vi "User jsObject.vi"(7 "DB Connection Ref":T1, 8 "error in (no error)":errorcluster, 9 "User Record (empty)":T2, 10 "User jsObject Name (\"USER\")":string="USER", 11 "Previous String (\"\")":string) -> (0 "error out":errorcluster, 2 "User Literal Object":string, 3 "User jsObject":string, 5 "User jsObject Definition":string)   [LabVIEW 2011]
uses:
  User Record.ctl
  SI.LIB/ODBC/SQL Controls/Connection Refnum.ctl
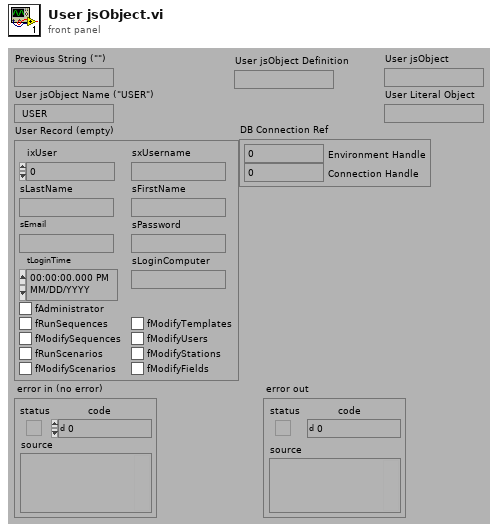
[diagram p1: front panel]
types:
  T1 = typedef "Connection Refnum.ctl" = cluster{"Environment Handle":i32, "Connection Handle":i32}
  T2 = typedef "User Record.ctl" = cluster{"ixUser":i32, "sxUsername":string, "sLastName":string, "sFirstName":string, "sEmail":string, "sPassword":string, "tLoginTime":timestamp, "sLoginComputer":string, "fAdministrator":bool, "fRunSequences":bool, "fModifySequences":bool, "fRunScenarios":bool, "fModifyScenarios":bool, "fModifyTemplates":bool, "fModifyUsers":bool, "fModifyStations":bool, "fModifyFields":bool}
  T3 = typedef "Station Record.ctl" = cluster{"ixStation":i32, "sxStationId":string, "sIP":string, "fVerified":bool}
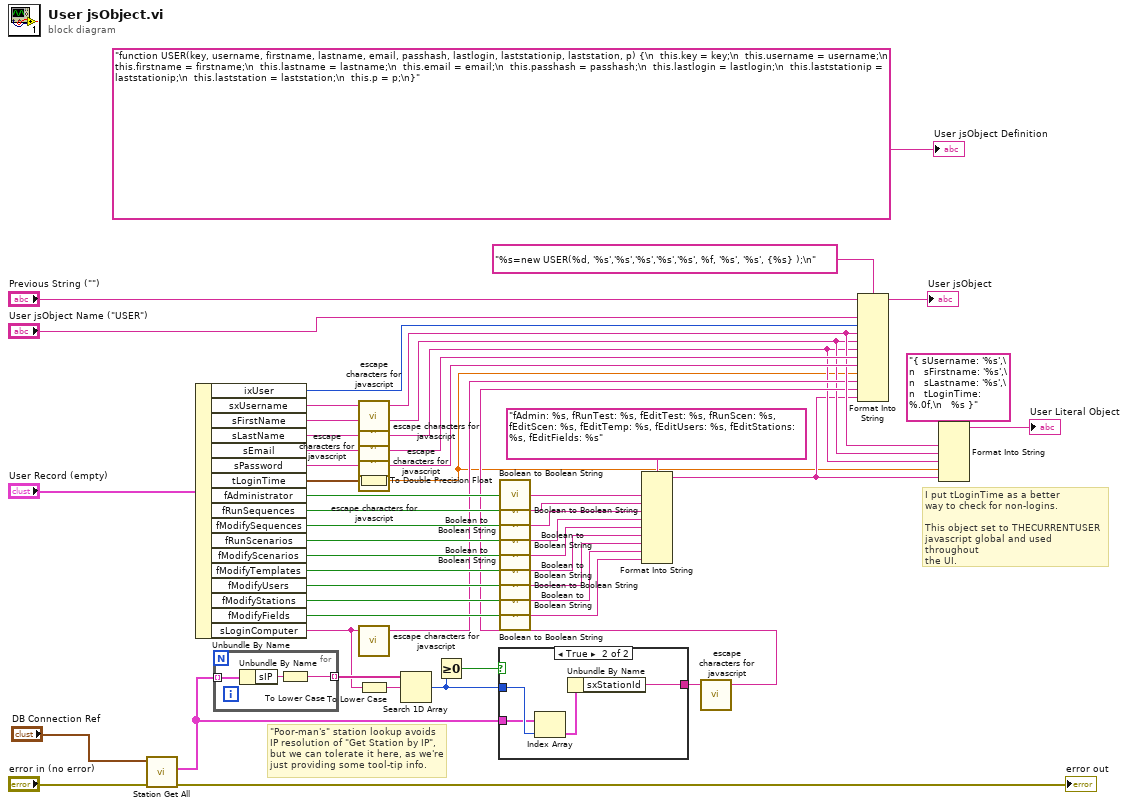
[diagram p0: block diagram]
diagram:
  # "I put tLoginTime as a better\nway to check for non-logins.\n\nThis object set to THECURRENTUSER\njavascript global and used throughout\nthe UI."
  # "\"Poor-man's\" station lookup avoids\nIP resolution of \"Get Station by IP\",\nbut we can tolerate it here, as we're\njust providing some tool-tip info."
  n1 = call "Station Get All.vi"("error in (no error)"="error in (no error)", "Connection Refnum"="DB Connection Ref") -> ("error out"=→"error out":errorcluster, "Station Records"=w38:T3[])  [unwired: 2 in, 6 out]
  n2 = Unbundle By Name("User Record (empty)") -> ("ixUser"=w23:i32, "sxUsername"=w32:string, "sFirstName"=w31:string, "sLastName"=w30:string, "sEmail"=w29:string, "sPassword"=w28:string, "tLoginTime"=w45:timestamp, "fAdministrator"=w52:bool, "fRunSequences"=w51:bool, "fModifySequences"=w50:bool, "fRunScenarios"=w49:bool, "fModifyScenarios"=w48:bool, "fModifyTemplates"=w47:bool, "fModifyUsers"=w46:bool, "fModifyStations"=w34:bool, "fModifyFields"=w33:bool, "sLoginComputer"=w27:string)
  n3 = for {
    tunnel: [w55] -> w37 mode=indexing
    tunnel: w38 -> [w54] mode=indexing
    n4 = Unbundle By Name(w54) -> ("sIP"=w56:string)
    n5 = To Lower Case(string=w56) -> (all lower case string=w55:string)
  }
  n6 = call "escape characters for javascript.vi"("String (\"\")"=w32) -> ("escaped String"=w20:string)  [unwired: 4 out]
  n7 = call "escape characters for javascript.vi"("String (\"\")"=w31) -> ("escaped String"=w17:string)  [unwired: 4 out]
  n8 = call "escape characters for javascript.vi"("String (\"\")"=w30) -> ("escaped String"=w16:string)  [unwired: 4 out]
  n9 = call "escape characters for javascript.vi"("String (\"\")"=w29) -> ("escaped String"=w22:string)  [unwired: 4 out]
  n10 = call "escape characters for javascript.vi"("String (\"\")"=w28) -> ("escaped String"=w21:string)  [unwired: 4 out]
  n11 = To Double Precision Float(number=w45) -> (double precision float=w4:dbl)
  n12 = call "escape characters for javascript.vi"("String (\"\")"=w27) -> ("escaped String"=w19:string)  [unwired: 4 out]
  n13 = To Lower Case(string=w27) -> (all lower case string=w42:string)
  n14 = Search 1D Array(1D array=w37, element=w42) -> (index of element=w40:i32)  [unwired: 1 out]
  n15 = Greater Or Equal To 0?(x=w40) -> (x >= 0?=w41:bool)
  n16 = case shown="True" w41 {
    tunnel: w40 -> [_ w60]
    tunnel: w38 -> [_ w59]
    tunnel: [_ w57] -> w26
    frame False {
    }
    frame True {
      n17 = Index Array(array=w59, index=w60) -> (element=w58:T3)
      n18 = Unbundle By Name(w58) -> ("sxStationId"=w57:string)
    }
  }
  n19 = call "Boolean to Boolean String.vi"("Boolean"=w52) -> ("Boolean string"=w14:string)  [unwired: 1 in]
  n20 = call "Boolean to Boolean String.vi"("Boolean"=w51) -> ("Boolean string"=w13:string)  [unwired: 1 in]
  n21 = call "Boolean to Boolean String.vi"("Boolean"=w50) -> ("Boolean string"=w12:string)  [unwired: 1 in]
  n22 = call "Boolean to Boolean String.vi"("Boolean"=w49) -> ("Boolean string"=w11:string)  [unwired: 1 in]
  n23 = call "Boolean to Boolean String.vi"("Boolean"=w48) -> ("Boolean string"=w10:string)  [unwired: 1 in]
  n24 = call "Boolean to Boolean String.vi"("Boolean"=w47) -> ("Boolean string"=w9:string)  [unwired: 1 in]
  n25 = call "Boolean to Boolean String.vi"("Boolean"=w46) -> ("Boolean string"=w8:string)  [unwired: 1 in]
  n26 = call "Boolean to Boolean String.vi"("Boolean"=w34) -> ("Boolean string"=w7:string)  [unwired: 1 in]
  n27 = call "Boolean to Boolean String.vi"("Boolean"=w33) -> ("Boolean string"=w6:string)  [unwired: 1 in]
  n28 = Format Into String(format string="fAdmin: %s, fRunTest: %s, fEditTest: %s, fRunScen: %s, fEditScen: %s, fEditTemp: %s, fEditUsers: %s, fEditStations: %s, fEditFields: %s", w14, w13, w12, w11, w10, w9, w8, w7, w6) -> (resulting string=w5:string)  [unwired: 2 in, 1 out]
  n29 = call "escape characters for javascript.vi"("String (\"\")"=w26) -> ("escaped String"=w18:string)  [unwired: 4 out]
  n30 = Format Into String(format string="%s=new USER(%d, '%s','%s','%s','%s','%s', %f, '%s', '%s', {%s} );\n", initial string="Previous String (\"\")", "User jsObject Name (\"USER\")", w23, w20, w17, w16, w22, w21, w4, w19, w18, w5) -> (resulting string=→"User jsObject":string)  [unwired: 1 in, 1 out]
  n31 = Format Into String(format string="{ sUsername: '%s',\n   sFirstname: '%s',\n   sLastname: '%s',\n   tLoginTime: %.0f,\n   %s }", w20, w17, w16, w4, w5) -> (resulting string=→"User Literal Object":string)  [unwired: 2 in, 1 out]
  "User jsObject Definition" <- "function USER(key, username, firstname, lastname, email, passhash, lastlogin, laststationip, laststation, p) {\n  this.key = key;\n  this.username = username;\n  this.firstname = firstname;\n  this.lastname = lastname;\n  this.email = email;\n  this.passhash = passhash;\n  this.lastlogin = lastlogin;\n  this.laststationip = laststationip;\n  this.laststation = laststation;\n  this.p = p;\n}"
